vi "Gerador_sinais_manual.vi"() -> ()   [LabVIEW 2020]
panel:
  out "Sine":dynamicdata(graph)
  in  "stop":bool
  in  "Fase":dbl(knob) scale=0.0..10.0
  in  "DC offset":dbl(knob) scale=0.0..10.0
  in  "Freqeuncia":dbl(knob) scale=0.0..500.0
  in  "Amplitude":dbl(knob) scale=0.0..10.0
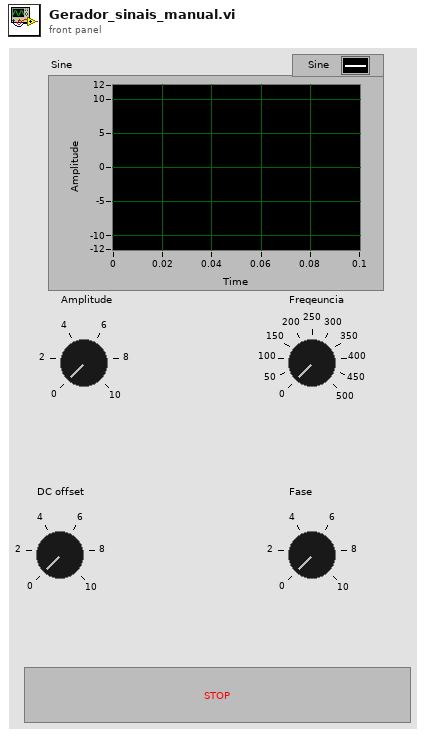
[diagram p1: front panel]
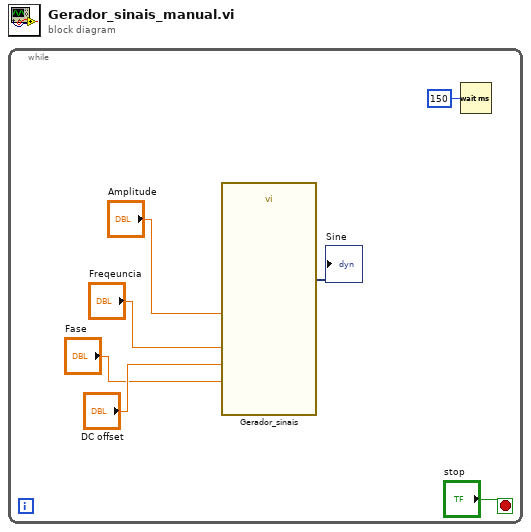
[diagram p0: block diagram]
diagram:
  n1 = while {
    stop <- "stop" stop-if-true
    n2 = call "Gerador_sinais.vi"("Offset"="DC offset", "Frequency"="Freqeuncia", "Amplitude"="Amplitude", "Phase"="Fase") -> ("Sine"=→"Sine":dynamicdata)  [unwired: 10 in, 1 out]
    n3 = Wait (ms)(milliseconds to wait=u32 150) -> ()  [unwired: 1 out]
  }
